vi "Brick.vi"(0 "Brick Ref table":refnum<vi>[](array[refnum]), 1 "HP set":i32[](array[numeric]), 2 "Hit Ref":refnum<vi>, 3 "Brick_ind":i32, 4 "Action":enum16{"Hit", "Set"}(ring)) -> (6 "Brick set":bool)   [LabVIEW 8.6]
uses:
  VI_Control/Brick Color Ctrl.ctl
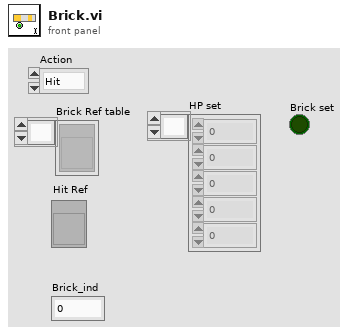
[diagram p1: front panel]
types:
  T1 = typedef "Brick Color Ctrl.ctl" = cluster{u32, u32}[][]
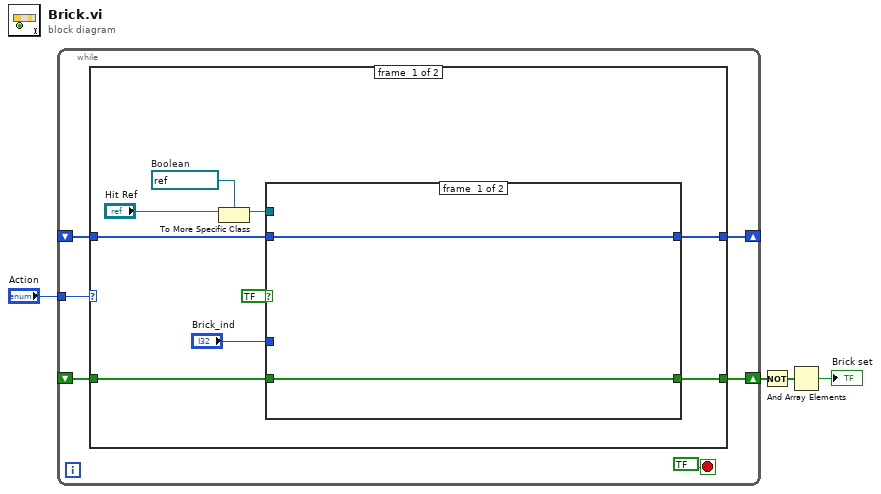
[diagram p0: block diagram]
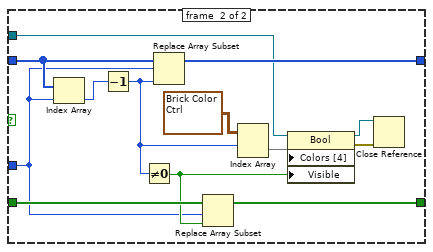
[diagram p2: hidden frame]
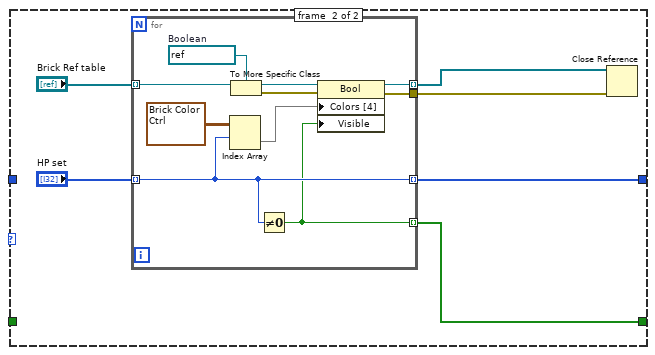
[diagram p3: hidden frame]
diagram:
  n1 = while {
    tunnel: "Action" -> [w9]
    shift-right: [w8] -> w2
    shift-left: _ -> [w6]
    shift-right: [w7] -> _
    shift-left: _ -> [w5]
    stop <- bool ? stop-if-true
    n2 = case shown="\"Set\"" w9 {
      tunnel: [w18 w38] -> w8
      tunnel: [w16 w37] -> w7
      tunnel: w6 -> [w19 _]
      tunnel: w5 -> [w17 _]
      frame #0 {
        w15 = refnum<vi> ?  # Boolean
        n3 = To More Specific Class(target class=w15, reference="Hit Ref") -> (specific class reference=w13:refnum<vi>)  [unwired: 1 in, 1 out]
        n4 = case shown="True" bool ? {
          tunnel: w19 -> [w20 w31]
          tunnel: [w20 w30] -> w18
          tunnel: w17 -> [w21 w29]
          tunnel: [w21 w28] -> w16
          tunnel: w13 -> [_ w27]
          tunnel: "Brick_ind" -> [_ w23]
          frame #0 {
          }
          frame #1 {
            n5 = Index Array(array=w29, index=w23) -> (element=w34:i32)
            n6 = Decrement(x=w34) -> (x-1=w26:i32)
            n7 = Not Equal To 0?(x=w26) -> (x != 0?=w25:bool)
            n8 = Replace Array Subset(array=w29, new element=w26, index=w23) -> (w28:i32[])
            n9 = Replace Array Subset(array=w31, new element=w25, index=w23) -> (w30:bool[])
            n10 = Index Array(array=T1 ? ("Colors [4]"), index (row)=w26) -> (element=w32:cluster{u32, u32}[])  [unwired: 1 in]
            n11 = property class="Bool"(reference=w27, "Colors [4]"=w32, "Visible"=w25) -> (reference out=w24:refnum<vi>, error out=w22:errorcluster)  [unwired: 1 in]
            n12 = Close Reference(reference=w24, error in (no error)=w22) -> ()  [unwired: 1 out]
          }
        }
      }
      frame #1 {
        n13 = for {
          tunnel: "HP set" -> [w44] mode=indexing
          tunnel: "Brick Ref table" -> [w47] mode=indexing
          tunnel: [w43] -> w38 mode=indexing
          tunnel: [w45] -> w36 mode=indexing
          tunnel: [w44] -> w37 mode=indexing
          tunnel: [w41] -> w35
          w48 = refnum<vi> ?  # Boolean
          n14 = Index Array(array=T1 ? ("Colors [4]"), index (row)=w44) -> (element=w50:cluster{u32, u32}[])  [unwired: 1 in]
          n15 = To More Specific Class(target class=w48, reference=w47) -> (specific class reference=w46:refnum<vi>, error out=w42:errorcluster)  [unwired: 1 in]
          n16 = Not Equal To 0?(x=w44) -> (x != 0?=w43:bool)
          n17 = property class="Bool"(reference=w46, error in=w42, "Colors [4]"=w50, "Visible"=w43) -> (reference out=w45:refnum<vi>, error out=w41:errorcluster)
        }
        n18 = Close Reference(reference=w36, error in (no error)=w35) -> ()  [unwired: 1 out]
      }
    }
  }
  n19 = Not(x=w2) -> (.not. x?=w3:bool[])
  n20 = And Array Elements(Boolean array=w3) -> (logical AND=→"Brick set":bool)
